vi "Autonomous Independent.vi"() -> ()   [LabVIEW 2013]
doc: "This VI is called when autonomous begins, and will automatically be terminated when autonomous ends. You can carry out timed or sensor driven robot movement independently without needing to return to the caller."
uses:
  <vilib>/Rock Robotics/WPI/Solenoid/WPI_SolenoidValue.ctl
  TargetType.ctl
  Robot Global Data.vi
  <vilib>/Rock Robotics/WPI/Solenoid/WPI_SolenoidSetEnum.vi
  <vilib>/addons/control/pid/pid.llb/PID (DBL).vi
  <vilib>/Rock Robotics/WPI/RobotDrive/WPI_RobotDriveArcadeDrive_Standard(NoSaturation).vi
  <vilib>/Rock Robotics/WPI/RobotDrive/WPI_RobotDriveGetSetRefNum.vi
  <vilib>/Rock Robotics/WPI/Joystick/WPI_JoystickGetSetRefNum.vi
  <vilib>/addons/control/pid/NI_PID_pid.lvlib
panel:
  in  "Drive Forward Time":u32=2000
  in  "Shoot Time":u32=1000
  out "4? (t)":bool
  out "Position":T1
  in  "Launcher State":enum16{"Shoot", "Out", "Retract"}(ring)
  in  "Shooter Extended Time":u32=500
  out "Shooter Tick":u32
  in  "Check Target Time":u32=500
  out "Left?":bool
  in  "Raise Arms Time":u32=1500
  in  "Up Position":dbl format="%.2f"
  in  "Close Arms Time":u32=250
  in  "Lower Arms Time":u32=1500
  in  "Down Position":dbl format="%.2f"
  in  "Open Arms Time":u32=250
  in  "Auton State":T2(ring)
  out "Tick at start of Auton":u32
  out "Current Movement, for debugging":T3 {"Y Joystick Value" scale=1.0..-1.0; "X Joystick Value" scale=-1.0..1.0}
  in  "Array of robot movements":T4(array[cluster]) {"Y Joystick Value" scale=1.0..-1.0; "X Joystick Value" scale=-1.0..1.0}
  # "Be sure to right-click and choose Data Operations>>Make Current Value default if you want to save the array values with the VI"
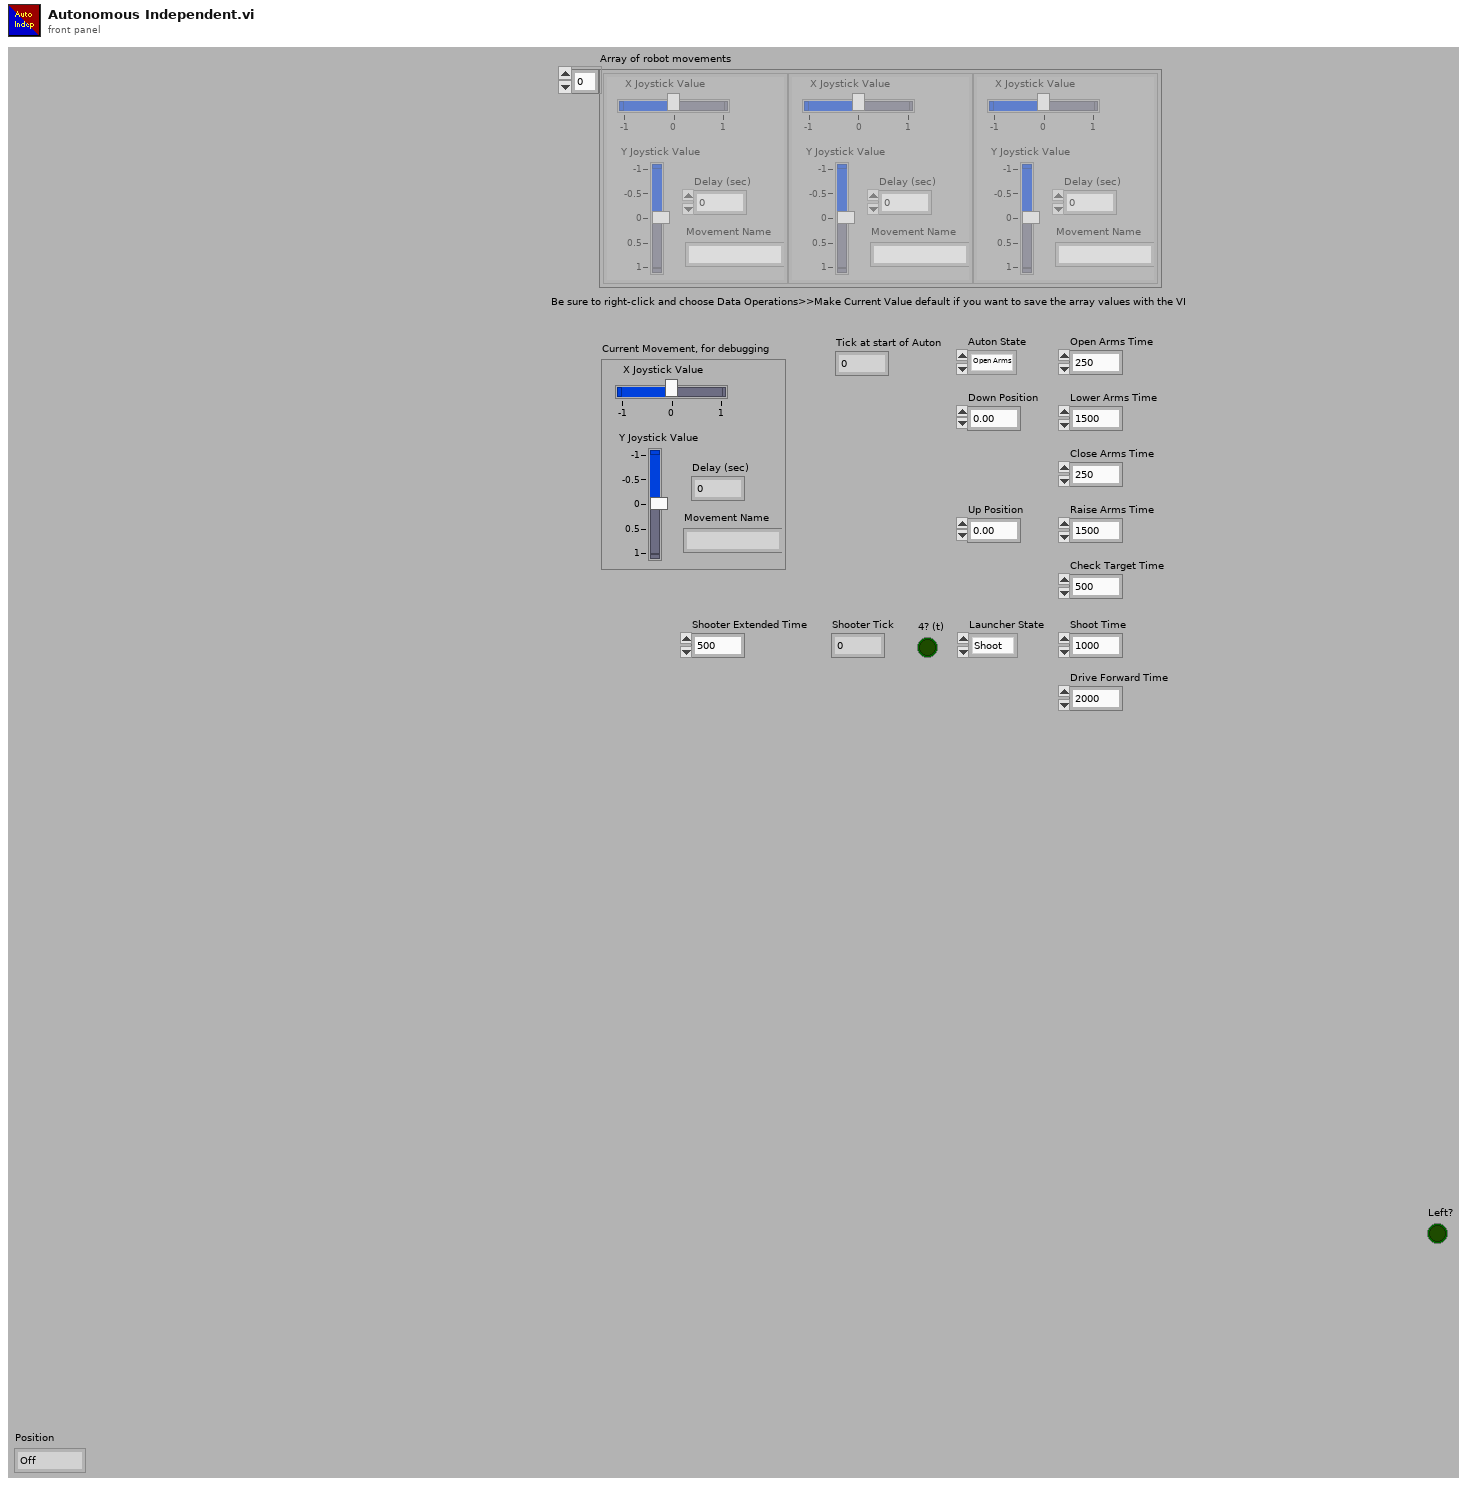
[diagram p1: front panel]
types:
  T1 = typedef "WPI_SolenoidValue.ctl" = enum16{"Off", "On", "Forward", "Reverse"}
  T2 = enum16{"Open Arms", "Lower Arms", "Close Arms", "Raise Arms", "Check Target", "Shoot", "Drive Forward", "Stop"}
  T3 = cluster{"X Joystick Value":dbl, "Y Joystick Value":dbl, "Delay (sec)":dbl, "Movement Name":string}
  T4 = cluster{"X Joystick Value":dbl, "Y Joystick Value":dbl, "Delay (sec)":dbl, "Movement Name":string}[]
  T5 = typedef "WPI_JoystickDevRef.ctl" = cluster{"Device":T6}
  T6 = typedef "WPI_JoystickDeviceEnum.ctl" = enum16{"USB 1", "USB 2", "USB 3", "USB 4", "Kinect 1", "Kinect 2"}
  T7 = cluster{"axis 1 (x)":dbl, "axis 2 (y)":dbl, "axis 3 (throttle)":dbl, "axis 4":dbl, "axis 5":dbl, "axis 6":dbl}
  T8 = enum16{"Open Arms", "Lower Arms", "Close Arms", "Raise Arms", "Check Target", "Shoot", "Drive Forward"}
  T9 = cluster{"proportional gain (Kc)":dbl, "integral time (Ti, min)":dbl, "derivative time (Td, min)":dbl}
  T10 = typedef "TargetType.ctl" = enum16{"Not Hot", "Hot"}
  T11 = typedef "WPI_SolenoidDevRef.ctl" = cluster{"DevStatus":errorcluster, "Solenoid Module":T12, "Forward Solenoid Channel":T13, "Reverse Solenoid Channel":T13}
  T12 = typedef "FPGA_TypedefSolenoidModule.ctl" = enum16{"Solenoid Module 1", "Solenoid Module 2"}
  T13 = typedef "WPI_SolenoidChannel.ctl" = enum8{"Solenoid 1", "Solenoid 2", "Solenoid 3", "Solenoid 4", "Solenoid 5", "Solenoid 6", "Solenoid 7", "Solenoid 8", "Invalid"}
  T14 = typedef "WPI_AnalogChannelDevRef.ctl" = cluster{"DevStatus":errorcluster, "Analog Module":T15, "Analog Channel":T16}
  T15 = typedef "FPGA_TypedefAnalogModule.ctl" = enum16{"Analog Module 1", "Analog Module 2"}
  T16 = typedef "FPGA_AIChannel.ctl" = enum8{"AI 1", "AI 2", "AI 3", "AI 4", "AI 5", "AI 6", "AI 7", "AI 8", "Invalid"}
  T17 = typedef "WPI_DigitalInputDevRef.ctl" = cluster{"DevStatus":errorcluster, "DIO Channel":T18, "Digital Module":T19}
  T18 = typedef "FPGA_DIOChannel.ctl" = enum8{"DIO 1", "DIO 2", "DIO 3", "DIO 4", "DIO 5", "DIO 6", "DIO 7", "DIO 8", "DIO 9", "DIO 10", "DIO 11", "DIO 12", "DIO 13", "DIO 14", "Invalid"}
  T19 = typedef "FPGA_TypedefDigitalModule.ctl" = enum16{"Digital Module 1", "Digital Module 2"}
  T20 = typedef "WPI_MotorControlDeviceRef.ctl" = cluster{"DeviceStatus":errorcluster, "Type":enum16{"PWM", "CAN"}, "PWM":cluster{"Digital Module":T19, "PWM Channel":T21, "DeadBand":T22}, "CAN":cluster{"Device Number":u8, "Control Mode":T23, "Semaphore":T24, "Max Vout":dbl}, "Invert":bool, "TransformRef":T25, "InvTransformRef":T25}
  T21 = typedef "FPGA_DIOPWMChannel.ctl" = enum8{"PWM 1", "PWM 2", "PWM 3", "PWM 4", "PWM 5", "PWM 6", "PWM 7", "PWM 8", "PWM 9", "PWM 10", "Invalid"}
  T22 = typedef "WPI_PWMDeadband.ctl" = cluster{"Name":string, "maxPositivePwm":i32, "minPositivePwm":i32, "centerPwm":i32, "maxNegativePwm":i32, "minNegativePwm":i32, "angularRange":u16}
  T23 = typedef "WPI_CANJaguar_ControlMode.ctl" = enum8{"Percent VBus", "Current", "Speed", "Position", "Voltage"}
  T24 = typedef "Semaphore RefNum" = refnum<k1>
  T25 = typedef "WPI_PWMTransform_ConPane.ctl" = refnum<vi>
  T26 = cluster{"Distance (ft)":dbl, "Target Center (-1 to 1)":cluster{"X":dbl, "Y":dbl}, "Left":bool, "State":T10}
  T27 = typedef "WPI_RobotDriveDevRef.ctl" = cluster{"DevStatus":errorcluster, "Motors[]":T20[], "Square Inputs":bool, "Max Output":dbl, "Isochronous":bool}
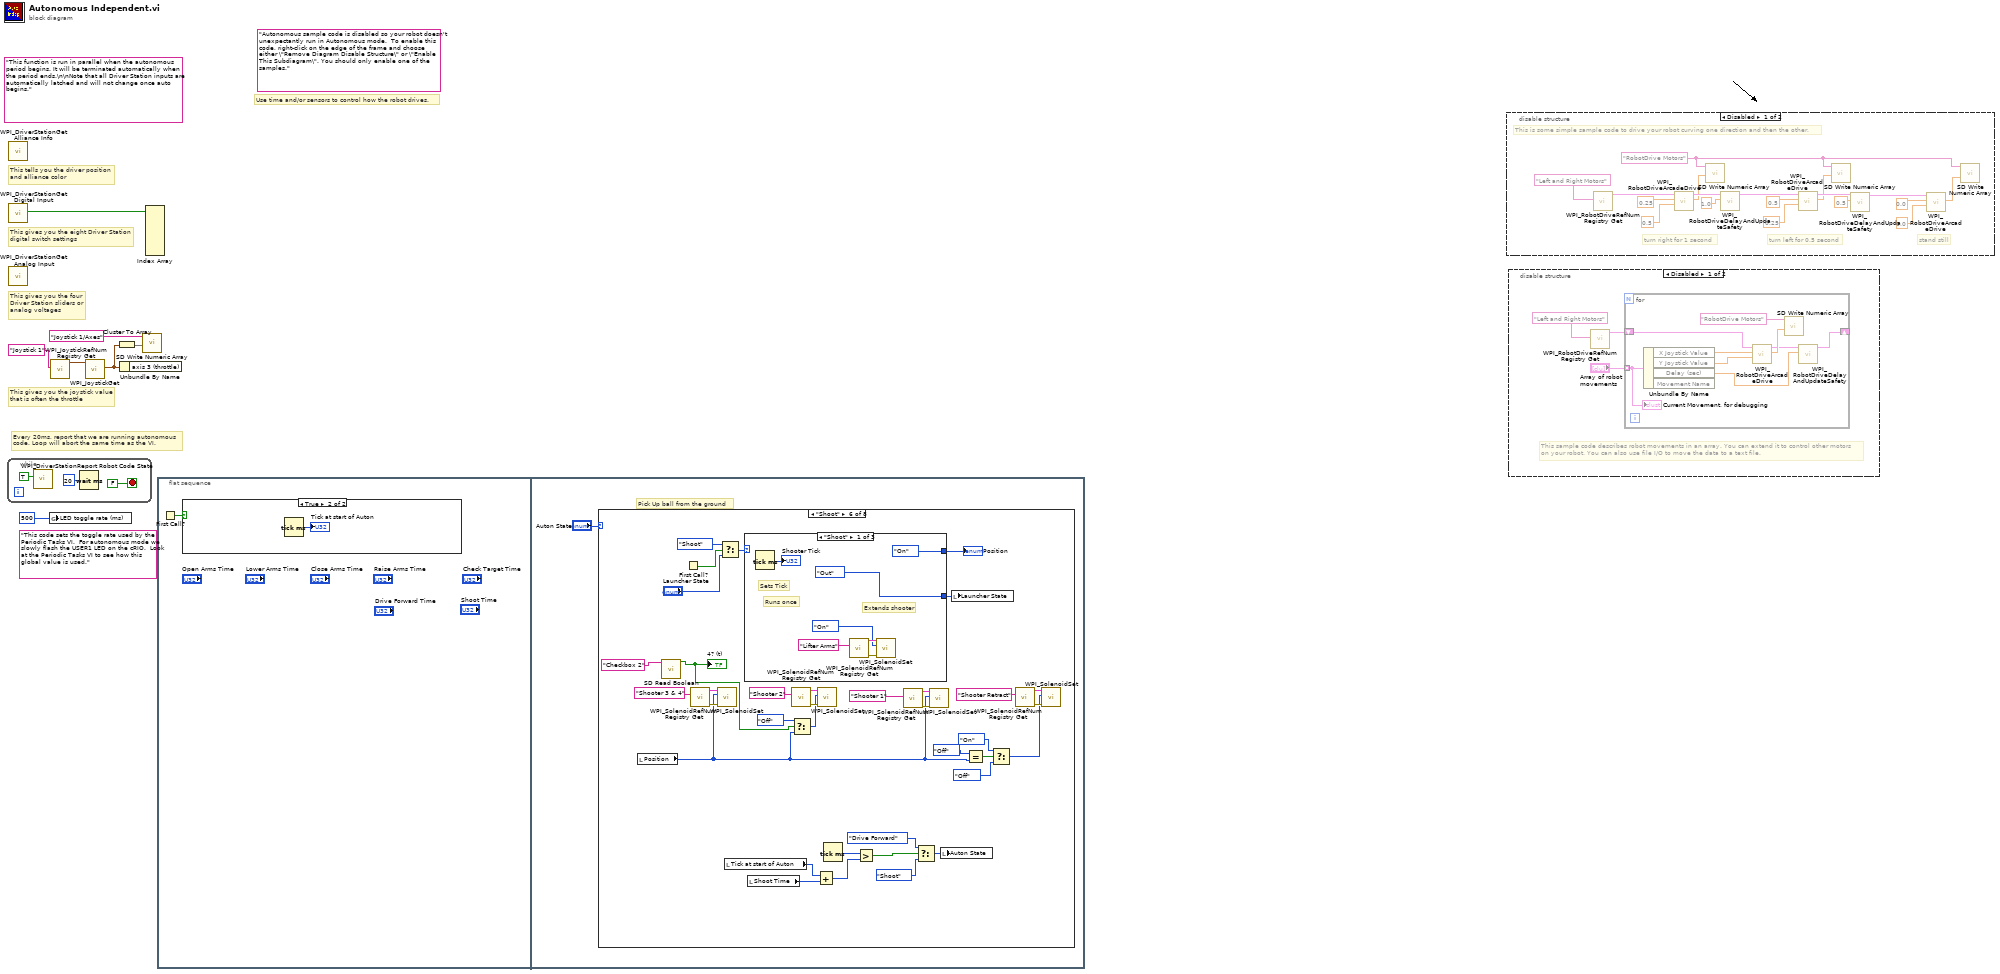
[diagram p0: block diagram]
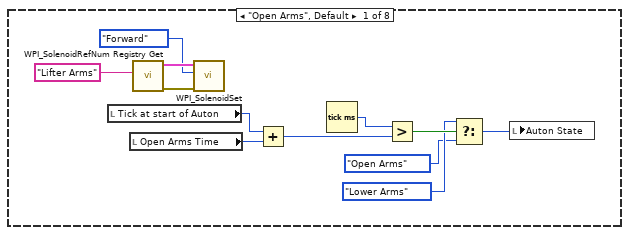
[diagram p3: hidden frame]
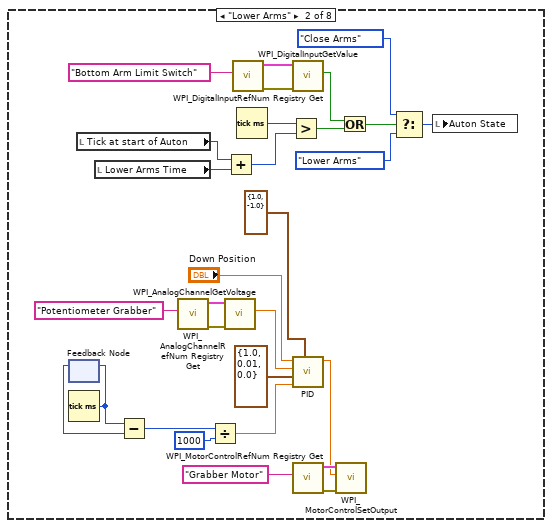
[diagram p4: hidden frame]
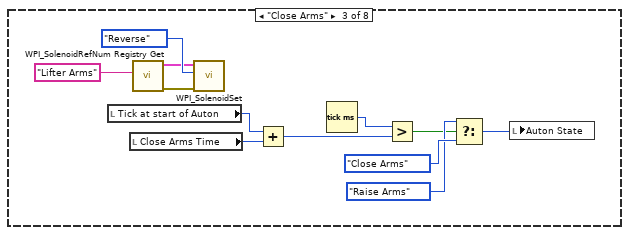
[diagram p5: hidden frame]
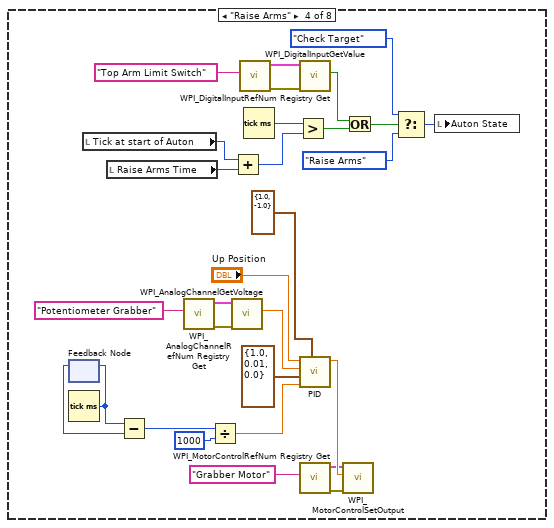
[diagram p6: hidden frame]
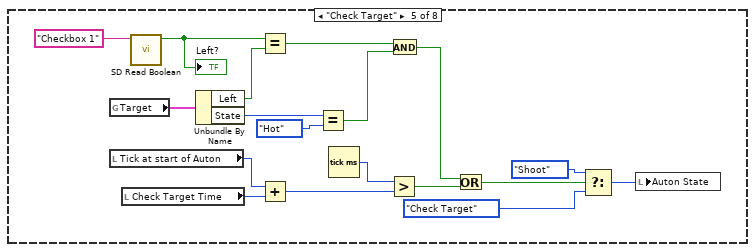
[diagram p7: hidden frame]
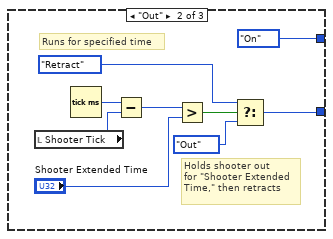
[diagram p8: hidden frame]
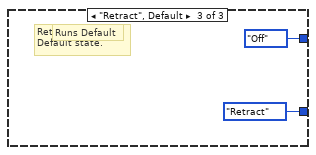
[diagram p9: hidden frame]
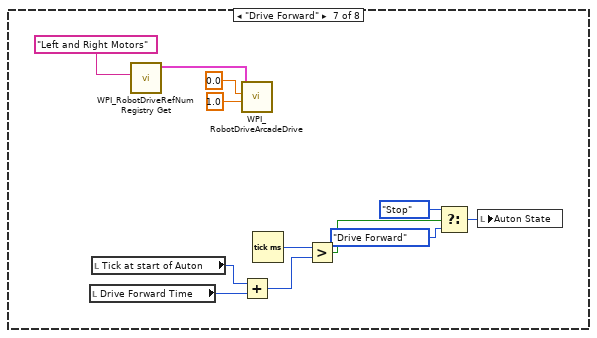
[diagram p10: hidden frame]
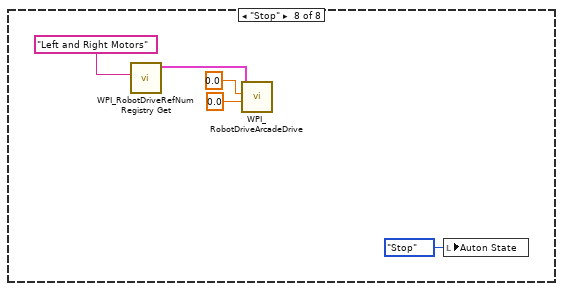
[diagram p11: hidden frame]
diagram:
  (unwired) "This code sets the toggle rate used by the Periodic Tasks VI.  For autonomous mode we slowly flash the USER1 LED on the cRIO.  Look at the Periodic Tasks VI to see how this global value is used."
  (unwired) "Autonomous sample code is disabled so your robot doesn't unexpectantly run in Autonomous mode.  To enable this code, right-click on the edge of the frame and choose either \"Remove Diagram Disable Structure\" or \"Enable This Subdiagram\". You should only enable one of the samples."
  (unwired) "This function is run in parallel when the autonomous period begins. It will be terminated automatically when the period ends.\n\nNote that all Driver Station inputs are automatically latched and will not change once auto begins."
  # "Every 20ms, report that we are running autonomous\ncode. Loop will abort the same time as the VI."
  # "This gives you the joystick value\nthat is often the throttle"
  # "Use time and/or sensors to control how the robot drives."
  # "This tells you the driver position\nand alliance color"
  # "This gives you the eight Driver Station\ndigital switch settings"
  # "This gives you the four\nDriver Station sliders or\nanalog voltages"
  n1 = while {
    stop <- FALSE stop-if-true
    n2 = call <vilib>:"WPI_DriverStationReport Robot Code State.vi"("Autonomous"=TRUE) -> ()  [unwired: 10 in, 1 out]
    n3 = Wait (ms)(milliseconds to wait=u32 20) -> ()  [unwired: 1 out]
  }
  n4 = call <vilib>:"WPI_DriverStationGet Alliance Info.vi"() -> ()  [unwired: 12 out]
  n5 = call <vilib>:"WPI_DriverStationGet Digital Input.vi"() -> ("Driver Station Digital Input (1-8)"=w7:bool[])  [unwired: 11 out]
  n6 = call <vilib>:"WPI_DriverStationGet Analog Input.vi"() -> ()  [unwired: 12 out]
  n7 = global write "Robot Global Data.vi" "LED toggle rate (ms)"(u32 500 ("LED ms toggle rate")) -> ()
  n8 = call <vilib>:"WPI_JoystickRefNum Registry Get.vi"("refnum name"="Joystick 1") -> ("JoystickDevRef"=w5:T5)  [unwired: 1 in, 9 out]
  n9 = call <vilib>:"WPI_JoystickGet.vi"("JoystickDevRef"=w5) -> ("Axes"=w2:T7)  [unwired: 1 in, 5 out]
  n10 = Cluster To Array(cluster=w2) -> (array=w3:dbl[])
  n11 = Unbundle By Name(w2) -> ()  [unwired: 1 out]
  n12 = call <vilib>:"SD Write Numeric Array.vi"("Numeric Array"=w3, "Name"="Joystick 1/Axes") -> ()  [unwired: 8 in, 2 out]
  n13 = Index Array(array=w7) -> ()  [unwired: 8 in, 8 out]
  n14 = flat-sequence {
    frame #0 {
      n15 = First Call?() -> (First Call?: T/F=w11:bool)
      n16 = case shown="True" w11 {
        frame False {
        }
        frame True {
          n17 = Tick Count (ms)() -> (millisecond timer value=→"Tick at start of Auton":u32)
        }
      }
    }
    frame #1 {
      # "Pick Up ball from the ground"
      n18 = case shown="\"Shoot\"" "Auton State" {
        frame "Open Arms", Default {
          n19 = local read "Tick at start of Auton"() -> (w19:u32)
          n20 = local read "Open Arms Time"() -> (w14:u32)
          n21 = call <vilib>:"WPI_SolenoidRefNum Registry Get.vi"("refnum name"="Lifter Arms") -> ("error out"=w24:errorcluster, "SolenoidDevRef"=w23:T11)  [unwired: 9 in]
          n22 = call-poly <vilib>:"WPI_SolenoidSet.vi"("error in (no error)"=w24, "Value"=WPI_SolenoidValue."Forward", "SolenoidDevRef"=w23) -> ()  [unwired: 7 in, 2 out]
          n23 = Add(x=w19, y=w14) -> (x+y=w18:u32)
          n24 = Tick Count (ms)() -> (millisecond timer value=w20:u32)
          n25 = Greater?(x=w20, y=w18) -> (0:w17:bool)
          n26 = Select(t=T8."Lower Arms", s=w17, f=T8."Open Arms") -> (s? t:f=w21:T8)
          n27 = local write "Auton State"(w21) -> ()
        }
        frame "Lower Arms" {
          n28 = feedback #1() -> (w49:u32)  [unwired: 1 in]
          n29 = Tick Count (ms)() -> (millisecond timer value=w50:u32)
          n30 = feedback-in #1(w50) -> ()
          n31 = local read "Tick at start of Auton"() -> (w31:u32)
          n32 = local read "Lower Arms Time"() -> (w29:u32)
          n33 = Subtract(x=w50, y=w49) -> (x-y=w48:u32)
          n34 = call <vilib>:"WPI_AnalogChannelRefNum Registry Get.vi"("refnum name"="Potentiometer Grabber") -> ("error out"=w52:errorcluster, "AIDeviceRef"=w53:T14)  [unwired: 9 in]
          n35 = Divide(x=w48, y=u32 1000) -> (x/y=w46:dbl)
          n36 = call <vilib>:"WPI_AnalogChannelGetVoltage.vi"("error in (no error)"=w52, "AIDeviceRef"=w53) -> ("Voltage"=w40:dbl)  [unwired: 7 in, 2 out]
          n37 = Add(x=w31, y=w29) -> (x+y=w30:u32)
          n38 = call <vilib>:"WPI_DigitalInputRefNum Registry Get.vi"("refnum name"="Bottom Arm Limit Switch") -> ("error out"=w35:errorcluster, "DigitalInputDevRef"=w34:T17)  [unwired: 9 in]
          n39 = Tick Count (ms)() -> (millisecond timer value=w32:u32)
          n40 = Greater?(x=w32, y=w30) -> (0:w26:bool)
          n41 = call <vilib>:"WPI_DigitalInputGetValue.vi"("error in (no error)"=w35, "DigitalInputDevRef"=w34) -> ("Value"=w27:bool)  [unwired: 7 in, 2 out]
          n42 = call-poly <vilib>:"PID.vi"("output range"=cluster{"output high":dbl, "output low":dbl} {"output high"=1.0, "output low"=-1.0}, "dt (s)"=w46, "PID gains"=T9 {"proportional gain (Kc)"=1.0, "integral time (Ti, min)"=0.01, "derivative time (Td, min)"=0.0}, "process variable"=w40, "setpoint"="Down Position") -> ("output"=w43:dbl)  [unwired: 5 in, 1 out]
          n43 = call <vilib>:"WPI_MotorControlRefNum Registry Get.vi"("refnum name"="Grabber Motor") -> ("error out"=w45:errorcluster, "MotorControlDevRef"=w44:T20)  [unwired: 9 in]
          n44 = call <vilib>:"WPI_MotorControlSetOutput.vi"("error in (no error)"=w45, "Output"=w43, "MotorControlDevRef"=w44) -> ()  [unwired: 6 in, 3 out]
          n45 = Or(x=w27, y=w26) -> (x .or. y?=w28:bool)
          n46 = Select(t=T8."Close Arms", s=w28, f=T8."Lower Arms") -> (s? t:f=w38:T8)
          n47 = local write "Auton State"(w38) -> ()
        }
        frame "Close Arms" {
          n48 = local read "Tick at start of Auton"() -> (w61:u32)
          n49 = local read "Close Arms Time"() -> (w66:u32)
          n50 = call <vilib>:"WPI_SolenoidRefNum Registry Get.vi"("refnum name"="Lifter Arms") -> ("error out"=w56:errorcluster, "SolenoidDevRef"=w57:T11)  [unwired: 9 in]
          n51 = call-poly <vilib>:"WPI_SolenoidSet.vi"("error in (no error)"=w56, "Value"=WPI_SolenoidValue."Reverse", "SolenoidDevRef"=w57) -> ()  [unwired: 7 in, 2 out]
          n52 = Add(x=w61, y=w66) -> (x+y=w62:u32)
          n53 = Tick Count (ms)() -> (millisecond timer value=w60:u32)
          n54 = Greater?(x=w60, y=w62) -> (0:w63:bool)
          n55 = Select(t=T8."Raise Arms", s=w63, f=T8."Close Arms") -> (s? t:f=w59:T8)
          n56 = local write "Auton State"(w59) -> ()
        }
        frame "Raise Arms" {
          n57 = feedback #2() -> (w72:u32)  [unwired: 1 in]
          n58 = Tick Count (ms)() -> (millisecond timer value=w71:u32)
          n59 = feedback-in #2(w71) -> ()
          n60 = local read "Tick at start of Auton"() -> (w90:u32)
          n61 = local read "Raise Arms Time"() -> (w92:u32)
          n62 = Subtract(x=w71, y=w72) -> (x-y=w73:u32)
          n63 = call <vilib>:"WPI_AnalogChannelRefNum Registry Get.vi"("refnum name"="Potentiometer Grabber") -> ("error out"=w69:errorcluster, "AIDeviceRef"=w68:T14)  [unwired: 9 in]
          n64 = Divide(x=w73, y=u32 1000) -> (x/y=w75:dbl)
          n65 = call <vilib>:"WPI_AnalogChannelGetVoltage.vi"("error in (no error)"=w69, "AIDeviceRef"=w68) -> ("Voltage"=w81:dbl)  [unwired: 7 in, 2 out]
          n66 = Add(x=w90, y=w92) -> (x+y=w91:u32)
          n67 = call <vilib>:"WPI_DigitalInputRefNum Registry Get.vi"("refnum name"="Top Arm Limit Switch") -> ("error out"=w86:errorcluster, "DigitalInputDevRef"=w87:T17)  [unwired: 9 in]
          n68 = Tick Count (ms)() -> (millisecond timer value=w89:u32)
          n69 = Greater?(x=w89, y=w91) -> (0:w95:bool)
          n70 = call <vilib>:"WPI_DigitalInputGetValue.vi"("error in (no error)"=w86, "DigitalInputDevRef"=w87) -> ("Value"=w94:bool)  [unwired: 7 in, 2 out]
          n71 = call-poly <vilib>:"PID.vi"("output range"=cluster{"output high":dbl, "output low":dbl} {"output high"=1.0, "output low"=-1.0}, "dt (s)"=w75, "PID gains"=T9 {"proportional gain (Kc)"=1.0, "integral time (Ti, min)"=0.01, "derivative time (Td, min)"=0.0}, "process variable"=w81, "setpoint"="Up Position") -> ("output"=w78:dbl)  [unwired: 5 in, 1 out]
          n72 = call <vilib>:"WPI_MotorControlRefNum Registry Get.vi"("refnum name"="Grabber Motor") -> ("error out"=w76:errorcluster, "MotorControlDevRef"=w77:T20)  [unwired: 9 in]
          n73 = call <vilib>:"WPI_MotorControlSetOutput.vi"("error in (no error)"=w76, "Output"=w78, "MotorControlDevRef"=w77) -> ()  [unwired: 6 in, 3 out]
          n74 = Or(x=w94, y=w95) -> (x .or. y?=w93:bool)
          n75 = Select(t=T8."Check Target", s=w93, f=T8."Raise Arms") -> (s? t:f=w83:T8)
          n76 = local write "Auton State"(w83) -> ()
        }
        frame "Check Target" {
          n77 = global read "Robot Global Data.vi" "Target"() -> (w113:T26)
          n78 = local read "Tick at start of Auton"() -> (w101:u32)
          n79 = local read "Check Target Time"() -> (w103:u32)
          n80 = call <vilib>:"SD Read Boolean.vi"("Name"="Checkbox 1" ("refnum name")) -> ("Boolean"=w108:bool)  [unwired: 8 in, 2 out]
          "Left?" <- w108
          n81 = Unbundle By Name(w113) -> ("Left"=w109:bool, "State"=w112:T10)
          n82 = Equal?(x=w108, y=w109) -> (x = y?=w106:bool)
          n83 = Add(x=w101, y=w103) -> (x+y=w102:u32)
          n84 = Equal?(x=w112, y=TargetType."Hot") -> (x = y?=w107:bool)
          n85 = Tick Count (ms)() -> (millisecond timer value=w100:u32)
          n86 = Greater?(x=w100, y=w102) -> (0:w105:bool)
          n87 = And(x=w106, y=w107) -> (x .and. y?=w96:bool)
          n88 = Or(x=w96, y=w105) -> (x .or. y?=w104:bool)
          n89 = Select(t=T8."Shoot", s=w104, f=T8."Check Target") -> (s? t:f=w97:T8)
          n90 = local write "Auton State"(w97) -> ()
        }
        frame "Shoot" {
          n91 = local read "Position"() -> (w126:T1)
          n92 = call <vilib>:"SD Read Boolean.vi"("Name"="Checkbox 2" ("refnum name")) -> ("Boolean"=w122:bool)  [unwired: 8 in, 2 out]
          "4? (t)" <- w122
          n93 = First Call?() -> (First Call?: T/F=w144:bool)
          n94 = call <vilib>:"WPI_SolenoidRefNum Registry Get.vi"("refnum name"="Shooter 3 & 4") -> ("error out"=w139:errorcluster, "SolenoidDevRef"=w138:T11)  [unwired: 9 in]
          n95 = call-poly <vilib>:"WPI_SolenoidSet.vi"("error in (no error)"=w139, "Value"=w126, "SolenoidDevRef"=w138) -> ()  [unwired: 7 in, 2 out]
          n96 = Select(t=enum16{"Shoot", "Out", "Retract"}."Shoot", s=w144, f="Launcher State") -> (s? t:f=w148:enum16{"Shoot", "Out", "Retract"})
          n97 = local read "Tick at start of Auton"() -> (w119:u32)
          n98 = case shown="\"Shoot\"" w148 {
            tunnel: [WPI_SolenoidValue."On" ("Value") WPI_SolenoidValue."On" ("Value") WPI_SolenoidValue."Off" ("Value")] -> w145
            tunnel: [enum16{"Shoot", "Out", "Retract"}."Out" ("Launcher State") w158 enum16{"Shoot", "Out", "Retract"}."Retract" ("Launcher State")] -> w146
            frame "Shoot" {
              # "Runs once"
              # "Sets Tick"
              # "Extends shooter"
              n99 = Tick Count (ms)() -> (millisecond timer value=→"Shooter Tick":u32)
              n100 = call <vilib>:"WPI_SolenoidRefNum Registry Get.vi"("refnum name"="Lifter Arms") -> ("error out"=w152:errorcluster, "SolenoidDevRef"=w151:T11)  [unwired: 9 in]
              n101 = call-poly <vilib>:"WPI_SolenoidSet.vi"("error in (no error)"=w152, "Value"=WPI_SolenoidValue."On", "SolenoidDevRef"=w151) -> ()  [unwired: 7 in, 2 out]
            }
            frame "Out" {
              # "Runs for specified time"
              # "Holds shooter out\nfor \"Shooter Extended\nTime,\" then retracts"
              n102 = local read "Shooter Tick"() -> (w164:u32)
              n103 = Tick Count (ms)() -> (millisecond timer value=w165:u32)
              n104 = Subtract(x=w165, y=w164) -> (x-y=w163:u32)
              n105 = Greater?(x=w163, y="Shooter Extended Time") -> (0:w162:bool)
              n106 = Select(t=enum16{"Shoot", "Out", "Retract"}."Retract" ("Launcher State"), s=w162, f=enum16{"Shoot", "Out", "Retract"}."Out" ("Launcher State")) -> (s? t:f=w158:enum16{"Shoot", "Out", "Retract"})
            }
            frame "Retract", Default {
              # "Runs Default"
              # "Retracts Shooter, \nDefault state."
            }
          }
          "Position" <- w145
          n107 = local read "Shoot Time"() -> (w121:u32)
          n108 = call <vilib>:"WPI_SolenoidRefNum Registry Get.vi"("refnum name"="Shooter 2") -> ("error out"=w142:errorcluster, "SolenoidDevRef"=w143:T11)  [unwired: 9 in]
          n109 = Select(t=WPI_SolenoidValue."Off", s=w122, f=w126) -> (s? t:f=w125:T1)
          n110 = Add(x=w119, y=w121) -> (x+y=w120:u32)
          n111 = call-poly <vilib>:"WPI_SolenoidSet.vi"("error in (no error)"=w142, "Value"=w125, "SolenoidDevRef"=w143) -> ()  [unwired: 7 in, 2 out]
          n112 = Tick Count (ms)() -> (millisecond timer value=w118:u32)
          n113 = Greater?(x=w118, y=w120) -> (0:w114:bool)
          n114 = call <vilib>:"WPI_SolenoidRefNum Registry Get.vi"("refnum name"="Shooter 1") -> ("error out"=w136:errorcluster, "SolenoidDevRef"=w135:T11)  [unwired: 9 in]
          n115 = Select(t=T8."Drive Forward", s=w114, f=T8."Shoot") -> (s? t:f=w116:T8)
          n116 = call-poly <vilib>:"WPI_SolenoidSet.vi"("error in (no error)"=w136, "Value"=w126, "SolenoidDevRef"=w135) -> ()  [unwired: 7 in, 2 out]
          n117 = local write "Auton State"(w116) -> ()
          n118 = local write "Launcher State"(w146) -> ()
          n119 = Equal?(x=WPI_SolenoidValue."Off", y=w126) -> (x = y?=w130:bool)
          n120 = Select(t=WPI_SolenoidValue."On" ("x"), s=w130, f=WPI_SolenoidValue."Off" ("x")) -> (s? t:f=w127:T1)
          n121 = call <vilib>:"WPI_SolenoidRefNum Registry Get.vi"("refnum name"="Shooter Retract") -> ("error out"=w133:errorcluster, "SolenoidDevRef"=w134:T11)  [unwired: 9 in]
          n122 = call-poly <vilib>:"WPI_SolenoidSet.vi"("error in (no error)"=w133, "Value"=w127, "SolenoidDevRef"=w134) -> ()  [unwired: 7 in, 2 out]
        }
        frame "Drive Forward" {
          n123 = local read "Drive Forward Time"() -> (w175:u32)
          n124 = local read "Tick at start of Auton"() -> (w173:u32)
          n125 = call <vilib>:"WPI_RobotDriveRefNum Registry Get.vi"("refnum name"="Left and Right Motors") -> ("RobotDriveDevRef"=w176:T27)  [unwired: 1 in, 9 out]
          n126 = call-poly <vilib>:"WPI_RobotDriveArcadeDrive.vi"("Y axis value"=1.0, "X axis value"=0.0, "RobotDriveDevRef"=w176) -> ()  [unwired: 6 in, 3 out]
          n127 = Add(x=w173, y=w175) -> (x+y=w174:u32)
          n128 = Tick Count (ms)() -> (millisecond timer value=w172:u32)
          n129 = Greater?(x=w172, y=w174) -> (0:w170:bool)
          n130 = Select(t=T2."Stop" ("Auton State"), s=w170, f=T2."Drive Forward" ("Auton State")) -> (s? t:f=w171:T2)
          n131 = local write "Auton State"(w171) -> ()
        }
        frame "Stop" {
          n132 = call <vilib>:"WPI_RobotDriveRefNum Registry Get.vi"("refnum name"="Left and Right Motors") -> ("RobotDriveDevRef"=w181:T27)  [unwired: 1 in, 9 out]
          n133 = call-poly <vilib>:"WPI_RobotDriveArcadeDrive.vi"("Y axis value"=0.0, "X axis value"=0.0, "RobotDriveDevRef"=w181) -> ()  [unwired: 6 in, 3 out]
          n134 = local write "Auton State"(T2."Stop" ("Auton State")) -> ()
        }
      }
    }
  }
  n135 = disable-structure shown="Disabled" {
    frame Disabled {
      w185 = "RobotDrive Motors" ("Name")
      # "This is some simple sample code to drive your robot curving one direction and then the other."
      # "stand still"
      # "turn left for 0.5 second"
      # "turn right for 1 second"
      n136 = call <vilib>:"WPI_RobotDriveRefNum Registry Get.vi"("refnum name"="Left and Right Motors") -> ("RobotDriveDevRef"=w189:T27)  [unwired: 1 in, 9 out]
      n137 = call-poly <vilib>:"WPI_RobotDriveArcadeDrive.vi"("Y axis value"=0.5 ("X axis value"), "X axis value"=0.25, "RobotDriveDevRef"=w189) -> ("Motor Values"=w188:dbl[], "RobotDriveDevRef"=w196:T27)  [unwired: 1 in, 6 out]
      n138 = call <vilib>:"SD Write Numeric Array.vi"("Numeric Array"=w188, "Name"=w185) -> ()  [unwired: 8 in, 2 out]
      n139 = call <vilib>:"WPI_RobotDriveDelayAndUpdateSafety.vi"("Delay (s)"=1.0, "RobotDriveDevRef"=w196) -> ("RobotDriveDevRef 2"=w195:T27)  [unwired: 8 in, 1 out]
      n140 = call-poly <vilib>:"WPI_RobotDriveArcadeDrive.vi"("Y axis value"=0.25 ("X axis value"), "X axis value"=0.5, "RobotDriveDevRef"=w195) -> ("Motor Values"=w187:dbl[], "RobotDriveDevRef"=w194:T27)  [unwired: 1 in, 6 out]
      n141 = call <vilib>:"SD Write Numeric Array.vi"("Numeric Array"=w187, "Name"=w185) -> ()  [unwired: 8 in, 2 out]
      n142 = call <vilib>:"WPI_RobotDriveDelayAndUpdateSafety.vi"("Delay (s)"=0.5, "RobotDriveDevRef"=w194) -> ("RobotDriveDevRef 2"=w193:T27)  [unwired: 8 in, 1 out]
      n143 = call-poly <vilib>:"WPI_RobotDriveArcadeDrive.vi"("Y axis value"=0.0 ("X axis value"), "X axis value"=0.0, "RobotDriveDevRef"=w193) -> ("Motor Values"=w186:dbl[])  [unwired: 1 in, 7 out]
      n144 = call <vilib>:"SD Write Numeric Array.vi"("Numeric Array"=w186, "Name"=w185) -> ()  [unwired: 8 in, 2 out]
    }
    frame Enabled {
    }
  }
  n145 = disable-structure shown="Disabled" {
    frame Disabled {
      # "This sample code describes robot movements in an array. You can extend it to control other motors\non your robot. You can also use file I/O to move the data to a text file."
      n146 = call <vilib>:"WPI_RobotDriveRefNum Registry Get.vi"("refnum name"="Left and Right Motors") -> ("RobotDriveDevRef"=w204:T27)  [unwired: 1 in, 9 out]
      n147 = for {
        shift-right: [w210] -> _
        shift-left: w204 -> [w211]
        tunnel: "Array of robot movements" -> [w206] mode=indexing
        n148 = Unbundle By Name(w206) -> ("X Joystick Value"=w209:dbl, "Y Joystick Value"=w208:dbl, "Delay (sec)"=w207:dbl)  [unwired: 1 out]
        n149 = call-poly <vilib>:"WPI_RobotDriveArcadeDrive.vi"("Y axis value"=w208, "X axis value"=w209, "RobotDriveDevRef"=w211) -> ("Motor Values"=w213:dbl[], "RobotDriveDevRef"=w212:T27)  [unwired: 1 in, 6 out]
        n150 = call <vilib>:"SD Write Numeric Array.vi"("Numeric Array"=w213, "Name"="RobotDrive Motors") -> ()  [unwired: 8 in, 2 out]
        n151 = call <vilib>:"WPI_RobotDriveDelayAndUpdateSafety.vi"("Delay (s)"=w207, "RobotDriveDevRef"=w212) -> ("RobotDriveDevRef 2"=w210:T27)  [unwired: 8 in, 1 out]
        "Current Movement, for debugging" <- w206
      }
    }
    frame Enabled {
    }
  }
